vi "Build Refresh Listbox Data.vi"(8 "error in":errorcluster, 10 "new ports":T3[](array[typedef])=[{"hardware channel"=0, "direction"=enum."Rx", "labels"=[]}, {"hardware channel"=0, "direction"=enum."Rx", "labels"=[]}], 11 "current ports":T3[](array[typedef])) -> (0 "error out":errorcluster, 3 "refresh listbox":T1[](array[typedef]))   [LabVIEW 2020, in "AIM ARINC 429 System Explorer.lvlib" / "Implementation.lvlib"]
uses:
  Implementation.lvlib
  Types/Refresh Symbols.ctl
  Types/Refresh Listbox.ctl
  Shared/Direction.ctl
  <vilib>/NI/NI VeriStand Encoding and Decoding/Encoding.ctl
  <vilib>/NI/NI VeriStand Encoding and Decoding/Encoding and Decoding.lvlib
  Shared/Parameter Definition.ctl
  Shared/VS Channel Definition for Parameter.ctl
  Shared/Transfer Type.ctl
  Shared/VS Channels Definition for Label.ctl
  Shared/VS Channels Definition for All Labels on Hardware Channel.ctl
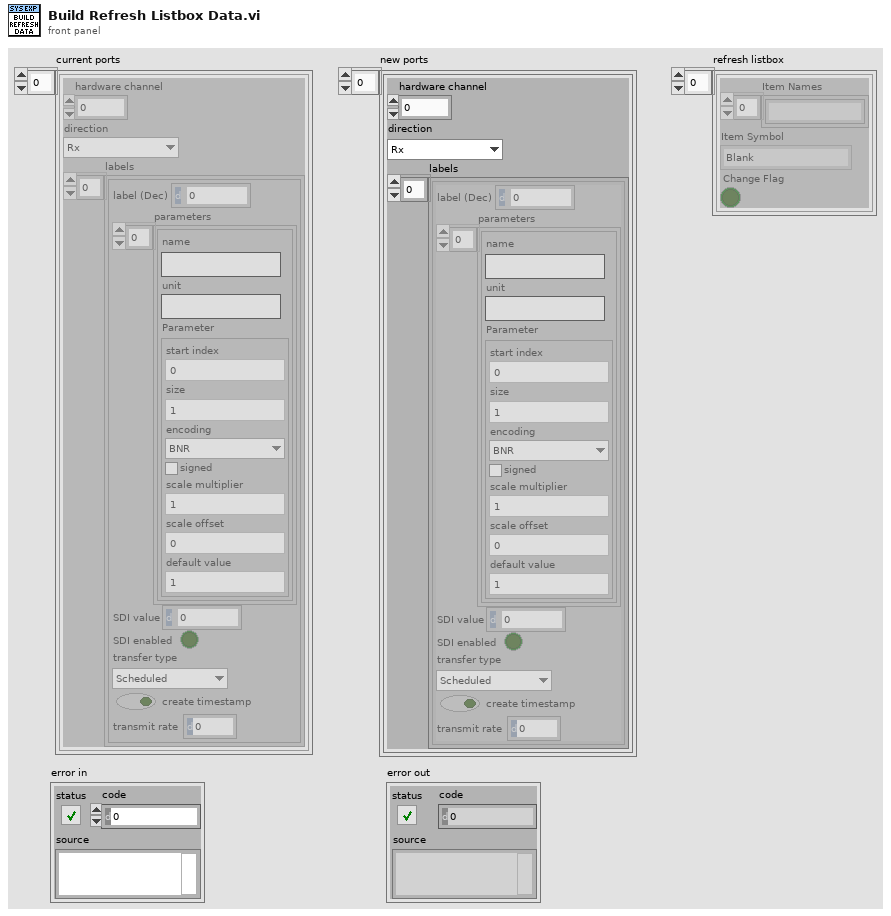
[diagram p1: front panel]
types:
  T1 = typedef "AIM ARINC 429 System Explorer.lvlib/Implementation.lvlib/Refresh Listbox.ctl" = cluster{"Item Names":string[], "Item Symbol":T2, "Change Flag":bool}
  T2 = typedef "AIM ARINC 429 System Explorer.lvlib/Implementation.lvlib/Refresh Symbols.ctl" = enum16{"Blank", "Port", "Incoming", "Outgoing", "Label", "Word", "Parameter", "ARINC-429", "Config Files", "Channel Spec", "Item"}
  T3 = typedef "VS Channels Definition for All Labels on Hardware Channel.ctl" = cluster{"hardware channel":i32, "direction":T4, "labels":T5[]}
  T4 = typedef "Direction.ctl" = enum16{"Rx", "Tx"}
  T5 = typedef "VS Channels Definition for Label.ctl" = cluster{"label (Dec)":u32, "parameters":T6[], "SDI value":u8, "SDI enabled":bool, "transfer type":T9, "create timestamp":bool, "transmit rate":u32}
  T6 = typedef "VS Channel Definition for Parameter.ctl" = cluster{"name":string, "unit":string, "Parameter":T7}
  T7 = typedef "Parameter Definition.ctl" = cluster{"start index":i32, "size":i32, "encoding":T8, "signed":bool, "scale multiplier":dbl, "scale offset":dbl, "default value":dbl}
  T8 = typedef "Encoding and Decoding.lvlib/Encoding.ctl" = enum16{"BNR", "BCD", "Discrete"}
  T9 = typedef "Transfer Type.ctl" = enum16{"Scheduled", "Acyclic", "Block", "Strobe"}
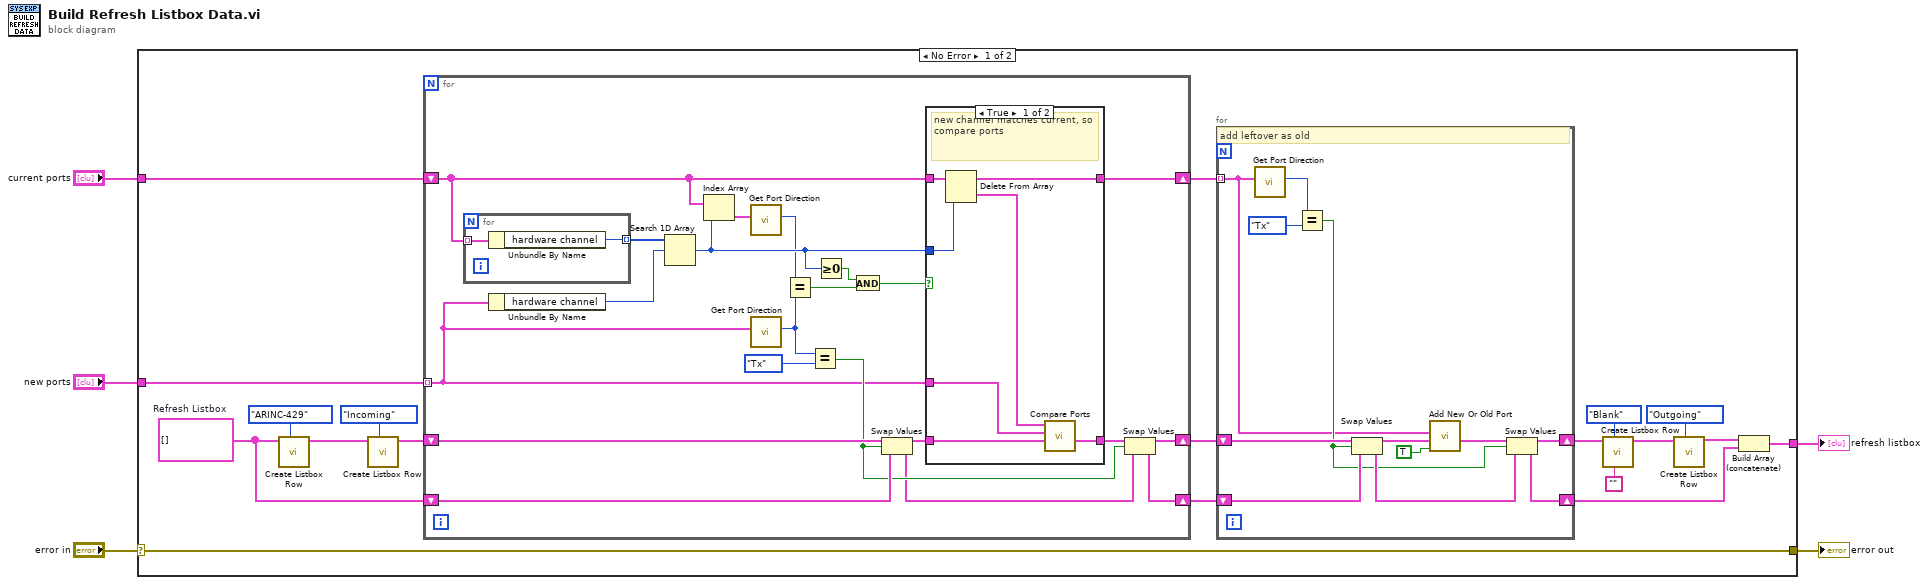
[diagram p0: block diagram]
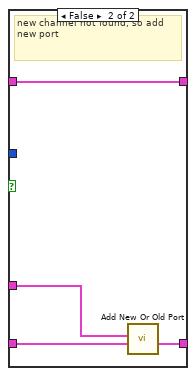
[diagram p2: hidden frame]
diagram:
  n1 = case shown="No Error" "error in" {
    selector: "error in" -> [w14 w71]
    tunnel: "new ports" -> [w24 _]
    tunnel: "current ports" -> [w23 _]
    tunnel: [w16 _] -> w3
    tunnel: [w14 w71] -> w1
    frame No Error {
      w15 = T1[] []  # Refresh Listbox
      n2 = call "Create Listbox Row.vi"("refresh symbol (Blank)"=Refresh_Symbols."ARINC-429" ("Refresh Symbol (Blank)"), "refresh listbox"=w15) -> ("refresh listbox out"=w17:T1[])  [unwired: 9 in]
      n3 = call "Create Listbox Row.vi"("refresh symbol (Blank)"=Refresh_Symbols."Incoming" ("Refresh Symbol (Blank)"), "refresh listbox"=w17) -> ("refresh listbox out"=w19:T1[])  [unwired: 9 in]
      n4 = for {
        tunnel: w24 -> [w38] mode=indexing
        shift-right: [w56] -> w6
        shift-left: w23 -> [w47]
        shift-right: [w55] -> w10
        shift-left: w19 -> [w52]
        shift-right: [w51] -> w8
        shift-left: w15 -> [w53]
        n5 = for {
          tunnel: w47 -> [w59] mode=indexing
          tunnel: [w58] -> w57 mode=indexing
          n6 = Unbundle By Name(w59) -> ("hardware channel"=w58:i32)
        }
        n7 = Unbundle By Name(w38) -> ("hardware channel"=w54:i32)
        n8 = Search 1D Array(1D array=w57, element=w54) -> (index of element=w46:i32)  [unwired: 1 in]
        n9 = Index Array(array=w47, index=w46) -> (element=w40:T3)
        n10 = call "Get Port Direction.vi"("port"=w40) -> ("direction"=w39:T4)  [unwired: 10 in]
        n11 = call "Get Port Direction.vi"("port"=w38) -> ("direction"=w37:T4)  [unwired: 10 in]
        n12 = Equal?(x=w39, y=w37) -> (x = y?=w49:bool)
        n13 = Equal?(x=w37, y=Direction."Tx" ("direction")) -> (x = y?=w44:bool)
        n14 = Greater Or Equal To 0?(x=w46) -> (x >= 0?=w50:bool)
        n15 = And(x=w50, y=w49) -> (x .and. y?=w48:bool)
        n16 = Swap Values(12:w52, 13:w44, 14:w53) -> (1:w43:T1[], 3:w42:T1[])
        n17 = case shown="True" w48 {
          tunnel: w47 -> [w66 w70]
          tunnel: [w65 w70] -> w56
          tunnel: w38 -> [w62 w67]
          tunnel: w43 -> [w63 w69]
          tunnel: [w64 w68] -> w41
          tunnel: w46 -> [w60 _]
          frame True {
            # "new channel matches current, so compare ports"
            n18 = Delete From Array(array=w66, index=w60) -> (deleted portion=w61:T3, array with subset deleted=w65:T3[])  [unwired: 1 in]
            n19 = call "Compare Ports.vi"("refresh listbox"=w63, "new port"=w62, "old port"=w61) -> ("refresh listbox out"=w64:T1[])  [unwired: 8 in]
          }
          frame False {
            # "new channel not found, so add new port"
            n20 = call "Add New Or Old Port.vi"("refresh listbox"=w69, "port"=w67) -> ("refresh listbox out"=w68:T1[])  [unwired: 9 in]
          }
        }
        n21 = Swap Values(12:w41, 13:w44, 14:w42) -> (1:w55:T1[], 3:w51:T1[])
      }
      n22 = for {
        shift-right: [w33] -> w9
        shift-left: w10 -> [w36]
        shift-right: [w30] -> w7
        shift-left: w8 -> [w32]
        tunnel: w6 -> [w26] mode=indexing
        # "add leftover as old"
        n23 = call "Get Port Direction.vi"("port"=w26) -> ("direction"=w25:T4)  [unwired: 10 in]
        n24 = Equal?(x=w25, y=Direction."Tx" ("direction")) -> (x = y?=w28:bool)
        n25 = Swap Values(12:w36, 13:w28, 14:w32) -> (1:w35:T1[], 3:w31:T1[])
        n26 = call "Add New Or Old Port.vi"("old port?"=TRUE, "refresh listbox"=w35, "port"=w26) -> ("refresh listbox out"=w34:T1[])  [unwired: 8 in]
        n27 = Swap Values(12:w34, 13:w28, 14:w31) -> (1:w33:T1[], 3:w30:T1[])
      }
      n28 = call "Create Listbox Row.vi"("override name"="", "refresh symbol (Blank)"=Refresh_Symbols."Blank" ("Refresh Symbol (Blank)"), "refresh listbox"=w9) -> ("refresh listbox out"=w11:T1[])  [unwired: 8 in]
      n29 = call "Create Listbox Row.vi"("refresh symbol (Blank)"=Refresh_Symbols."Outgoing" ("Refresh Symbol (Blank)"), "refresh listbox"=w11) -> ("refresh listbox out"=w21:T1[])  [unwired: 9 in]
      n30 = Build Array (concatenate)(w21, w7) -> (w16:T1[])
    }
    frame Error {
    }
  }
  "error out" <- w1
  "refresh listbox" <- w3
